vi "EnFlo_Error_Handler.vi"(3 "error in (no error)":errorcluster, 4 "Error Type":string, 5 "Dialog Box (T)":bool=TRUE) -> (0 "Continue":bool, 1 "SMS Message":string, 2 "Email Message":string)   [LabVIEW 2012]
uses:
  Controls/Post_Process.ctl
  <vilib>/Utility/error.llb/DialogType.ctl
  Globals/Meas_global.vi
  Globals/Trav_pos_global.vi
  Globals/Preference_global.vi
  Email_transfer_global.vi
  Globals/Dynamic_call_global.ph.vi
panel:
  out "error out":errorcluster
  in  "Case Constant\n(See Context Help)":bool
  out "Server copy Location":path
  out "Hours Running":dbl format="%.2f"
  out "Raw data file Local":path
  out "Error Information":string
  out "Log Files":path[](array[path])
  out "Frequency":i32
  out "Error Analysis":string
  out "Error Types":string[](array[string])
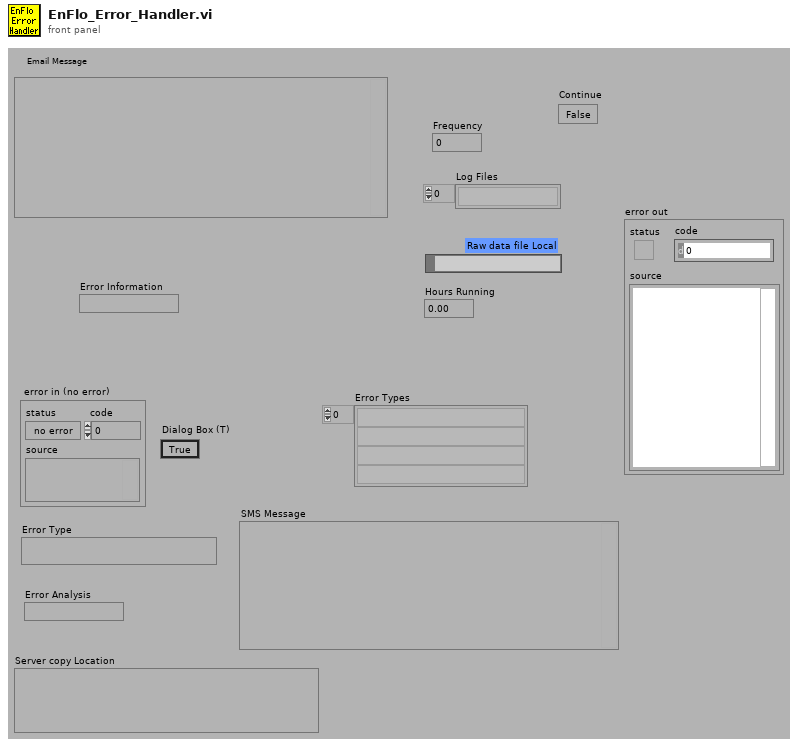
[diagram p1: front panel]
types:
  T1 = typedef "Post_Process.ctl" = enum16{"Take New Data", "Post Process Raw Data File"}
  T2 = cluster{"path":path, "data":string, "binary":bool, "MIME content-type \n(application/octet-stream)":string}[]
  T3 = typedef "DialogType.ctl" = u16
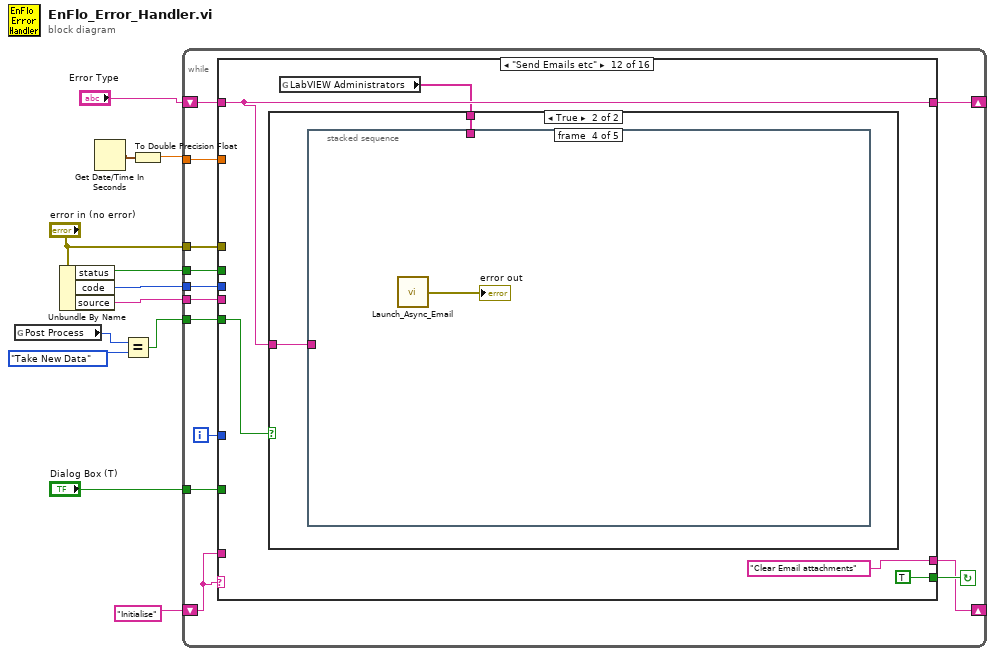
[diagram p0: block diagram]
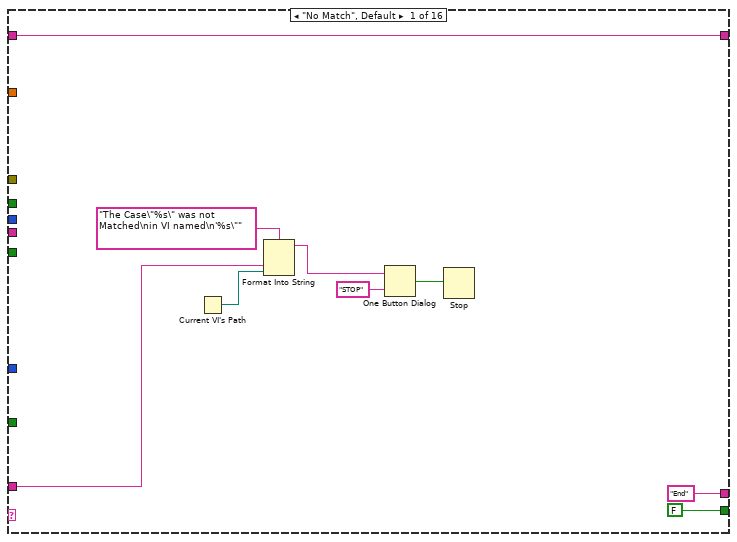
[diagram p2: hidden frame]
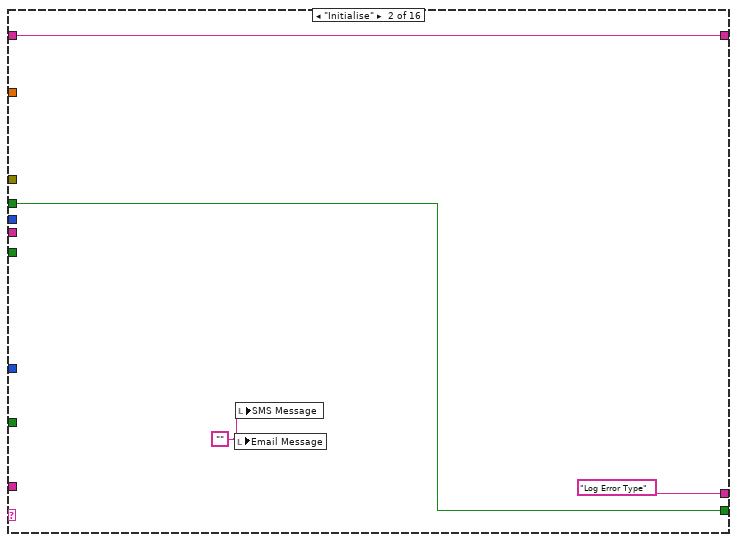
[diagram p3: hidden frame]
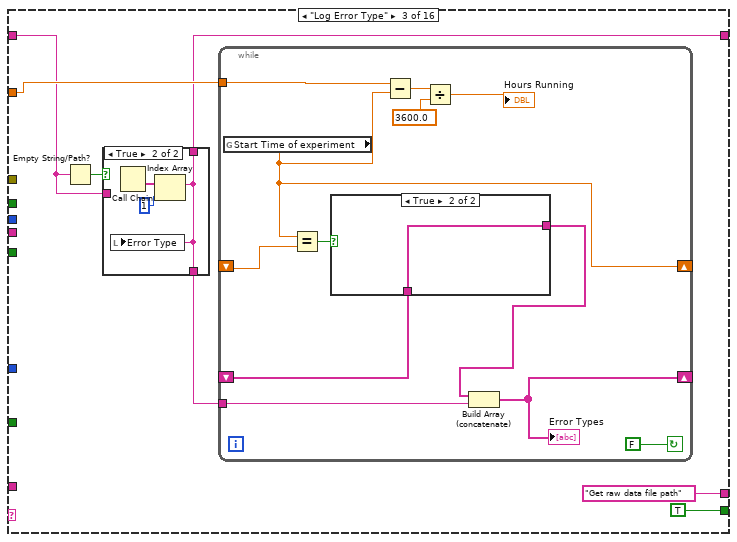
[diagram p4: hidden frame]
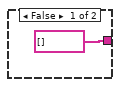
[diagram p5: hidden frame]
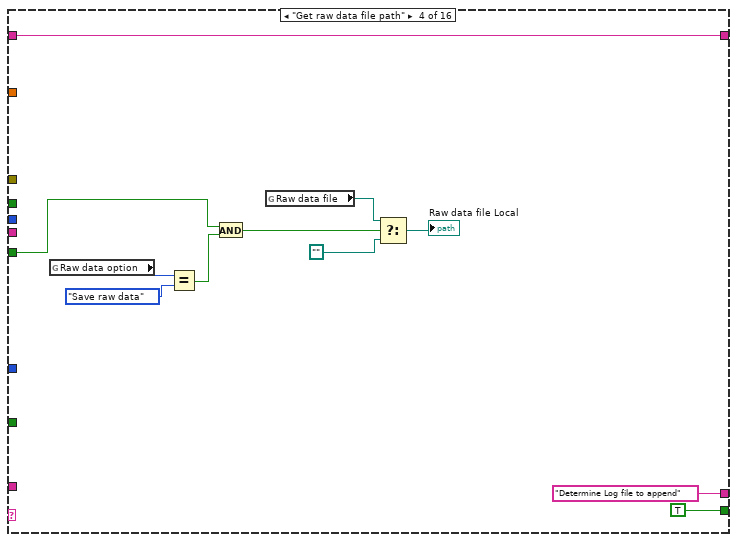
[diagram p7: hidden frame]
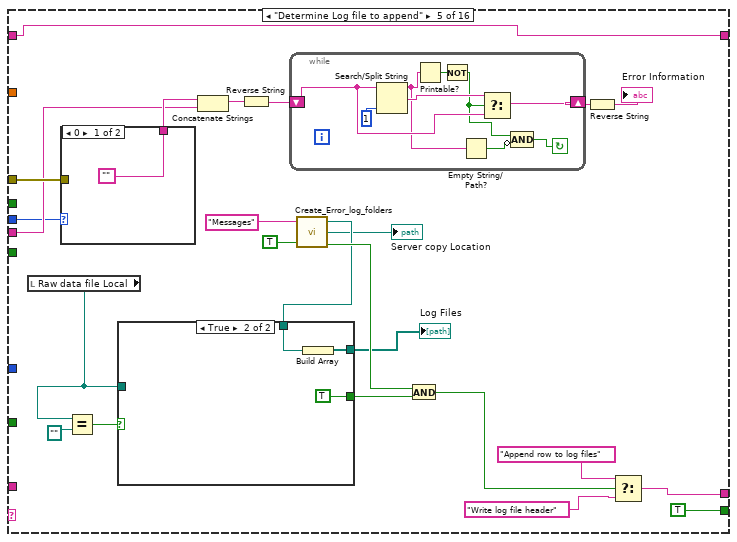
[diagram p8: hidden frame]
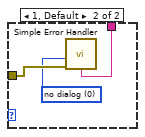
[diagram p9: hidden frame]
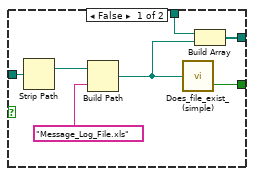
[diagram p10: hidden frame]
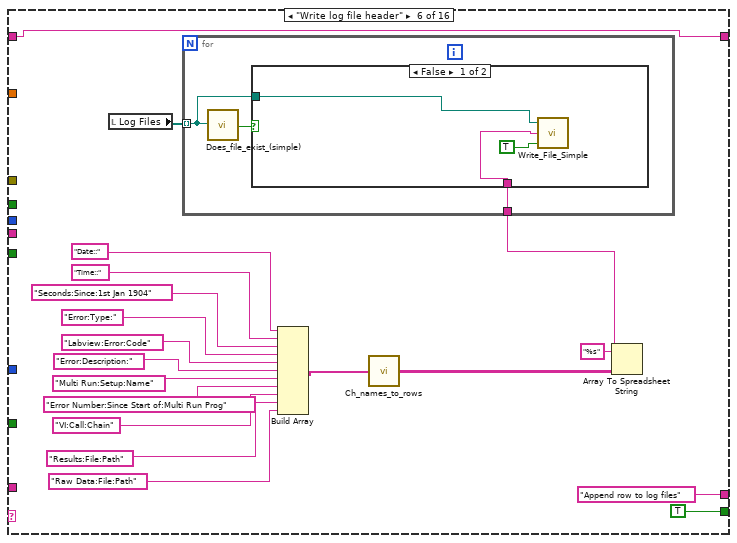
[diagram p11: hidden frame]
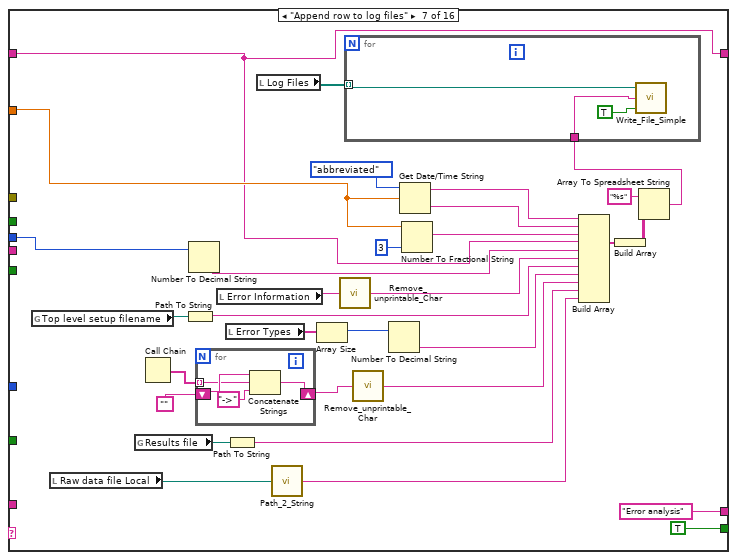
[diagram p13: hidden frame]
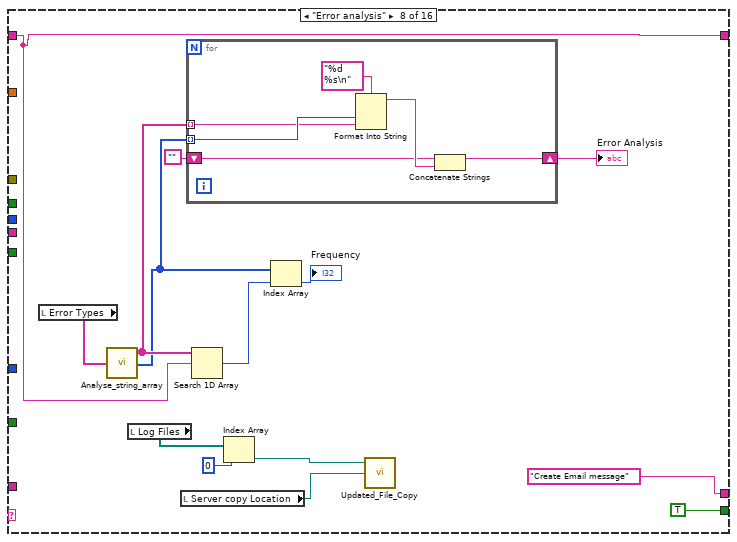
[diagram p14: hidden frame]
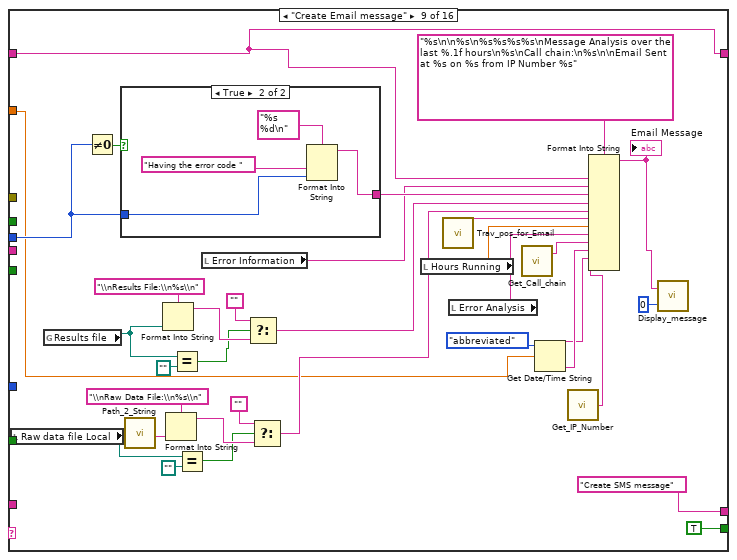
[diagram p15: hidden frame]
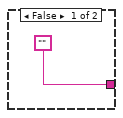
[diagram p16: hidden frame]
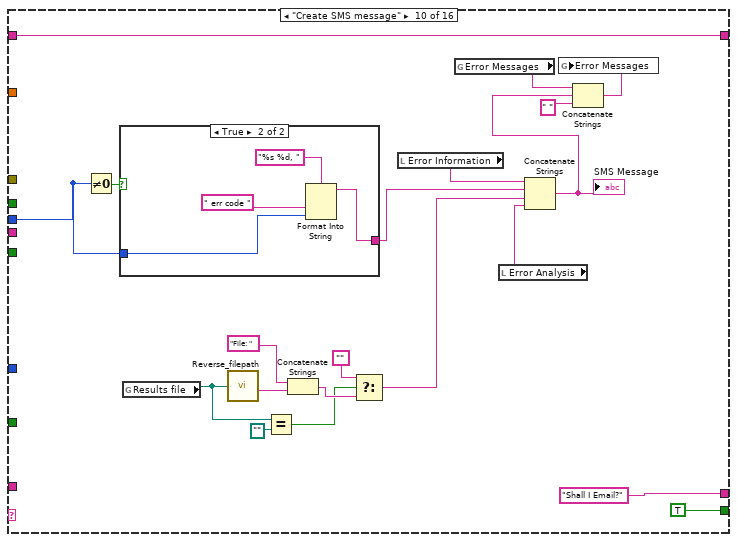
[diagram p17: hidden frame]
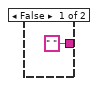
[diagram p18: hidden frame]
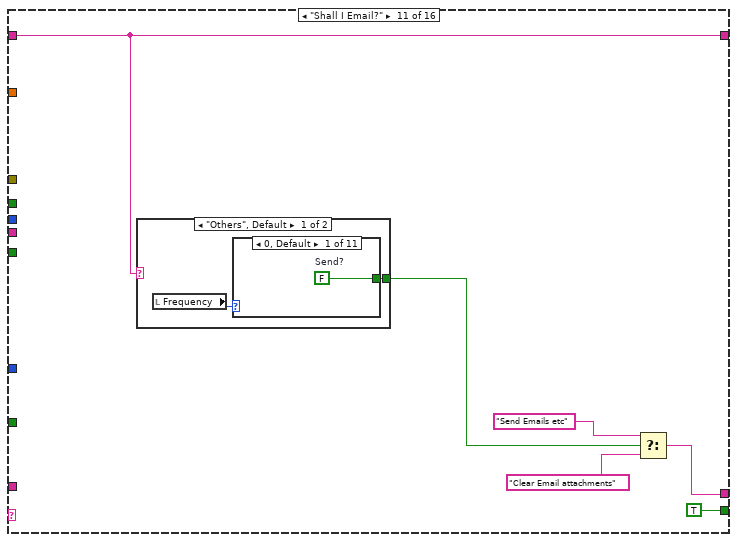
[diagram p19: hidden frame]
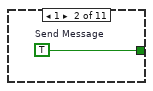
[diagram p20: hidden frame]
diagram:
  n1 = global read "Meas_global.vi" "Post Process"() -> (w5:T1)
  n2 = Unbundle By Name("error in (no error)") -> ("status"=w11:bool, "code"=w10:i32, "source"=w9:string)
  n3 = Get Date/Time In Seconds() -> (seconds since 1Jan1904=w8:timestamp)
  n4 = Equal?(x=w5, y=Post_Process."Take New Data" ("Post Process")) -> (x = y?=w3:bool)
  n5 = To Double Precision Float(number=w8) -> (double precision float=w12:dbl)
  n6 = while {
    tunnel: w9 -> [w19]
    tunnel: w10 -> [w21]
    tunnel: w11 -> [w22]
    tunnel: w12 -> [w23]
    shift-left: "Initialise" -> [w18]
    shift-right: [w24] -> _
    shift-right: [w16] -> _
    shift-left: "Error Type" -> [w17]
    tunnel: w3 -> [w15]
    tunnel: "Dialog Box (T)" -> [w14]
    tunnel: "error in (no error)" -> [w13]
    i -> [w20]
    stop <- w25 continue-if-true
    n7 = case shown="\"Send Emails etc\"" w18 {
      tunnel: [FALSE ("Abort") w38 TRUE ("status") TRUE ("status") TRUE ("status") TRUE TRUE TRUE ("status") TRUE ("Abort") TRUE ("status") TRUE ("Abort") TRUE ("Abort") TRUE ("Abort") w340 w351 FALSE ("Abort")] -> w25
      tunnel: ["End" ("f") "Log Error Type" "Get raw data file path" ("f") "Determine Log file to append" ("f") w96 "Append row to log files" ("f") "Error analysis" ("f") "Create Email message" ("f") "Create SMS message" "Shall I Email?" w272 "Clear Email attachments" "Is ADAM scan table running?" ("f") "Show timed error dialog" "Stop" "End"] -> w24
      tunnel: w23 -> [_ _ w42 _ _ _ w152 _ w215 _ _ _ _ _ _ _]
      tunnel: w22 -> [_ w38 _ _ _ _ _ _ _ _ _ _ _ _ _ _]
      tunnel: w21 -> [_ _ _ _ w75 _ w172 _ w237 w262 _ _ _ _ _ _]
      tunnel: w20 -> [_ _ _ _ _ _ _ _ _ _ _ _ _ _ _ _]
      tunnel: w19 -> [_ _ _ _ w77 _ _ _ _ _ _ _ _ _ _ _]
      tunnel: w18 -> [w29 _ _ _ _ _ _ _ _ _ _ _ _ _ _ _]
      tunnel: w17 -> [w26 w35 w40 w67 w82 w122 w149 w190 w209 w244 w274 w292 w338 w342 w349 w355]
      tunnel: [w26 w35 w39 w67 w82 w122 w149 w190 w209 w244 w274 w292 w338 w342 w349 w355] -> w16
      tunnel: w15 -> [_ _ _ w64 _ _ _ _ _ _ _ w289 _ _ _ _]
      tunnel: w14 -> [_ _ _ _ _ _ _ _ _ _ _ _ _ w339 _ _]
      tunnel: w13 -> [_ _ _ _ w79 _ _ _ _ _ _ _ _ _ _ _]
      frame "No Match", Default {
        n8 = Current VI's Path() -> (path=w30:path)
        n9 = Format Into String(format string="The Case\"%s\" was not Matched\nin VI named\n'%s\"" ("Format String"), w29, w30) -> (resulting string=w33:string)  [unwired: 2 in, 1 out]
        n10 = One Button Dialog(message=w33, button name ("OK")="STOP") -> (true=w31:bool)
        n11 = Stop(stop? (T)=w31) -> ()
      }
      frame "Initialise" {
        w37 = ""
        n12 = local write "Email Message"(w37) -> ()
        n13 = local write "SMS Message"(w37) -> ()
      }
      frame "Log Error Type" {
        n14 = Empty String/Path?(string/path=w40) -> (empty?=w44:bool)
        n15 = case shown="True" w44 {
          tunnel: [w60 w61] -> w43
          tunnel: w40 -> [w60 _]
          tunnel: [w60 w61] -> w39
          frame False {
          }
          frame True {
            n16 = Call Chain() -> (call chain=w63:string[])
            n17 = Index Array(array=w63, index=1 ("Index")) -> (element=w61:string)
            n18 = local write "Error Type"(w61) -> ()
          }
        }
        n19 = while {
          tunnel: w42 -> [w48]
          shift-left: _ -> [w55]
          shift-right: [w54] -> _
          shift-left: _ -> [w53]
          shift-right: [w51] -> _
          tunnel: w43 -> [w56]
          stop <- FALSE continue-if-true
          n20 = global read "Meas_global.vi" "Start Time of experiment"() -> (w51:dbl)
          n21 = Equal?(x=w51, y=w53) -> (x = y?=w52:bool)
          n22 = case shown="True" w52 {
            tunnel: [string[] [] w59] -> w57
            tunnel: w55 -> [_ w59]
            frame False {
            }
            frame True {
            }
          }
          n23 = Subtract(x=w48, y=w51) -> (x-y=w50:dbl)
          n24 = Divide(x=w50, y=3600.0) -> (x/y=→"Hours Running":dbl)
          n25 = Build Array (concatenate)(w57, w56) -> (w54:string[])
          "Error Types" <- w54
        }
      }
      frame "Get raw data file path" {
        n26 = global read "Meas_global.vi" "Raw data option"() -> (w73:enum16{"Save raw data", "Raw data not saved"})
        n27 = Equal?(x=w73, y=enum16{"Save raw data", "Raw data not saved"}."Save raw data" ("Raw data option")) -> (x = y?=w71:bool)
        n28 = And(x=w64, y=w71) -> (x .and. y?=w70:bool)
        n29 = global read "Meas_global.vi" "Raw data file"() -> (w66:path)
        n30 = Select(t=w66, s=w70, f=path "") -> (s? t:f=→"Raw data file Local":path)
      }
      frame "Determine Log file to append" {
        n31 = local read "Raw data file Local"() -> (w85:path)
        n32 = case shown="0" w75 {
          tunnel: w79 -> [_ w102]
          tunnel: ["" w100] -> w78
          frame 0 {
          }
          frame 1, Default {
            w101 = T3 0 items=["no dialog", "OK message", "continue or stop message", "OK message + warnings", "continue/stop + warnings"] ("type of dialog (OK msg:1)")
            n33 = call <vilib>:"Simple Error Handler.vi"("type of dialog (OK msg:1)"=w101, "error in (no error)"=w102) -> ("message"=w100:string)  [unwired: 7 out]
          }
        }
        n34 = Equal?(x=w85, y=path "") -> (x = y?=w94:bool)
        n35 = Concatenate Strings(w78, w77) -> (w76:string)
        n36 = Reverse String(1:w76) -> (0:w88:string)
        n37 = while {
          shift-left: w88 -> [w109]
          shift-right: [w108] -> w87
          stop <- w103 continue-if-true
          n38 = Search/Split String(string=w109, offset (0)=1 ("length")) -> (substring before match=w106:string, match + rest of string=w110:string)  [unwired: 2 out]
          n39 = Printable?(1:w106) -> (0:w107:bool)
          n40 = Not(x=w107) -> (.not. x?=w105:bool)
          n41 = Empty String/Path?(string/path=w106) -> (empty?=w104:bool)
          n42 = Select(t=w110, s=w105, f=w109) -> (s? t:f=w108:string)
          n43 = Compound Arithmetic op=AND(w105, invert w104) -> (w103:bool)
        }
        n44 = call "Create_Error_log_folders.vi"("Per Day Log File?"=TRUE, "Log Filename"="Messages" ("Input Element")) -> ("exists?"=w92:bool, "Server copy Location"=→"Server copy Location":path, "Local Log File"=w90:path)  [unwired: 1 in]
        n45 = case shown="True" w94 {
          tunnel: w85 -> [w118 _]
          tunnel: [w115 TRUE ("exists?")] -> w93
          tunnel: w90 -> [w114 w120]
          tunnel: [w112 w119] -> w89
          frame False {
            n46 = Strip Path(path=w118) -> (stripped path=w117:path)  [unwired: 1 out]
            n47 = Build Path(base path=w117, name or relative path="Message_Log_File.xls") -> (appended path=w113:path)
            n48 = call "Does_file_exist_(simple).vi"("Pathname"=w113) -> ("exists?"=w115:bool)
            n49 = Build Array(w114, w113) -> (w112:path[])
          }
          frame True {
            n50 = Build Array(w120) -> (w119:path[])
          }
        }
        "Log Files" <- w89
        n51 = And(x=w92, y=w93) -> (x .and. y?=w91:bool)
        n52 = Reverse String(1:w87) -> (0:→"Error Information":string)
        n53 = Select(t="Append row to log files", s=w91, f="Write log file header") -> (s? t:f=w96:string)
      }
      frame "Write log file header" {
        n54 = local read "Log Files"() -> (w126:path[])
        n55 = Build Array("Date::", "Time::", "Seconds:Since:1st Jan 1904", "Error:Type:", "Labview:Error:Code", "Error:Description:", "Multi Run:Setup:Name", "Error Number:Since Start of:Multi Run Prog", "VI:Call:Chain", "Results:File:Path", "Raw Data:File:Path") -> (w125:string[])
        n56 = call "Ch_names_to_rows.vi"("Channel Names"=w125) -> ("3 Row names"=w124:string[][])
        n57 = Array To Spreadsheet String(array=w124, 3:"%s" ("format string")) -> (spreadsheet string=w130:string)  [unwired: 1 out]
        n58 = for {
          tunnel: w130 -> [w143]
          tunnel: w126 -> [w141] mode=indexing
          n59 = call "Does_file_exist_(simple).vi"("Pathname"=w141) -> ("exists?"=w142:bool)
          n60 = case shown="False" w142 {
            tunnel: w143 -> [w145 _]
            tunnel: w141 -> [w144 _]
            frame False {
              n61 = call "Write_File_Simple.vi"("append to file? (new file:F)"=TRUE, "character string"=w145, "file path"=w144) -> ()  [unwired: 2 out]
            }
            frame True {
            }
          }
        }
      }
      frame "Append row to log files" {
        n62 = global read "Trav_pos_global.vi" "Top level setup filename"() -> (w174:path)
        n63 = local read "Raw data file Local"() -> (w148:path)
        n64 = global read "Meas_global.vi" "Results file"() -> (w157:path)
        n65 = Call Chain() -> (call chain=w162:string[])
        n66 = Path To String(path=w174) -> (string=w169:string)
        n67 = Number To Decimal String(number=w172) -> (decimal integer string=w171:string)  [unwired: 1 out]
        n68 = for {
          shift-right: [w181] -> w161
          shift-left: "" -> [w184]
          tunnel: w162 -> [w183] mode=indexing
          n69 = Concatenate Strings(w184, w183, "->" ("Substring")) -> (w181:string)
        }
        n70 = local read "Error Information"() -> (w154:string)
        n71 = local read "Error Types"() -> (w167:string[])
        n72 = Path To String(path=w157) -> (string=w156:string)
        n73 = local read "Log Files"() -> (w155:path[])
        n74 = call "Path_2_String.vi"("Real Path"=w148) -> ("Path String"=w147:string)
        n75 = Array Size(array=w167) -> (size(s)=w173:i32)
        n76 = call "Remove_unprintable_Char.vi"("Input String"=w154) -> ("Output String"=w170:string)
        n77 = call "Remove_unprintable_Char.vi"("Input String"=w161) -> ("Output String"=w163:string)
        n78 = Number To Decimal String(number=w173) -> (decimal integer string=w168:string)  [unwired: 1 out]
        n79 = Get Date/Time String(date format (0)=enum16{"short", "long", "abbreviated"}."abbreviated", seconds (now)=w152) -> (date string=w176:string, time string=w175:string)  [unwired: 1 out]
        n80 = Number To Fractional String(number=w152, precision (6)=i16 3) -> (F-format string=w151:string)  [unwired: 2 out]
        n81 = Build Array(w176, w175, w151, w149, w171, w170, w169, w168, w163, w156, w147) -> (w158:string[])
        n82 = Build Array(w158) -> (w166:string[][])
        n83 = Array To Spreadsheet String(array=w166, 3:"%s" ("format string")) -> (spreadsheet string=w164:string)  [unwired: 1 out]
        n84 = for {
          tunnel: w164 -> [w179]
          tunnel: w155 -> [w178] mode=indexing
          n85 = call "Write_File_Simple.vi"("append to file? (new file:F)"=TRUE, "character string"=w179, "file path"=w178) -> ()  [unwired: 2 out]
        }
      }
      frame "Error analysis" {
        n86 = local read "Error Types"() -> (w193:string[])
        n87 = call "Analyse_string_array.vi"("String array"=w193) -> ("Unique strings"=w197:string[], "Frequency"=w196:i32[])  [unwired: 1 out]
        n88 = local read "Log Files"() -> (w188:path[])
        n89 = local read "Server copy Location"() -> (w185:path)
        n90 = for {
          tunnel: w197 -> [w202] mode=indexing
          tunnel: w196 -> [w203] mode=indexing
          shift-right: [w199] -> w194
          shift-left: "" -> [w200]
          n91 = Format Into String(format string="%d %s\n" ("Format String"), w203, w202) -> (resulting string=w201:string)  [unwired: 2 in, 1 out]
          n92 = Concatenate Strings(w200, w201) -> (w199:string)
        }
        "Error Analysis" <- w194
        n93 = Search 1D Array(1D array=w197, element=w190) -> (index of element=w198:i32)  [unwired: 1 out]
        n94 = Index Array(array=w188, index=0) -> (element=w186:path)
        n95 = Index Array(array=w196, index=w198) -> (element=→"Frequency":i32)
        n96 = call "Updated_File_Copy.vi"("Target Path"=w185, "Source Path"=w186) -> ()  [unwired: 2 out]
      }
      frame "Create Email message" {
        n97 = local read "Raw data file Local"() -> (w206:path)
        n98 = global read "Meas_global.vi" "Results file"() -> (w222:path)
        n99 = Not Equal To 0?(x=w237) -> (x != 0?=w238:bool)
        n100 = case shown="True" w238 {
          tunnel: w237 -> [_ w242]
          tunnel: ["" w240] -> w236
          frame False {
          }
          frame True {
            n101 = Format Into String(format string="%s %d\n" ("Format String"), "Having the error code ", w242) -> (resulting string=w240:string)  [unwired: 2 in, 1 out]
          }
        }
        n102 = call "Path_2_String.vi"("Real Path"=w206) -> ("Path String"=w205:string)
        n103 = Format Into String(format string="\\nResults File:\\n%s\\n" ("Format String"), w222) -> (resulting string=w228:string)  [unwired: 2 in, 1 out]
        n104 = Format Into String(format string="\\nRaw Data File:\\n%s\\n" ("Format String"), w205) -> (resulting string=w226:string)  [unwired: 2 in, 1 out]
        n105 = Equal?(x=w222, y=path "") -> (x = y?=w221:bool)
        n106 = Equal?(x=w206, y=path "") -> (x = y?=w223:bool)
        n107 = local read "Error Information"() -> (w220:string)
        n108 = Select(t="", s=w221, f=w228) -> (s? t:f=w231:string)
        n109 = Select(t="", s=w223, f=w226) -> (s? t:f=w230:string)
        n110 = local read "Hours Running"() -> (w218:dbl)
        n111 = call "Trav_pos_for_Email.vi"() -> ("String"=w219:string)
        n112 = local read "Error Analysis"() -> (w217:string)
        n113 = call "Get_Call_chain.vi"() -> ("Output String"=w216:string)  [unwired: 1 in, 1 out]
        n114 = Get Date/Time String(date format (0)=enum16{"short", "long", "abbreviated"}."abbreviated", seconds (now)=w215) -> (date string=w211:string, time string=w213:string)  [unwired: 1 out]
        n115 = call "Get_IP_Number.vi"() -> ("IP Number"=w207:string)
        n116 = Format Into String(format string="%s\n\n%s\n%s%s%s%s\nMessage Analysis over the last %.1f hours\n%s\nCall chain:\n%s\n\nEmail Sent at %s on %s from IP Number %s" ("Format String"), w209, w220, w236, w231, w230, w219, w218, w217, w216, w213, w211, w207) -> (resulting string=w212:string)  [unwired: 2 in, 1 out]
        "Email Message" <- w212
        n117 = call "Display_message.vi"("Time to display message"=u32 0, "Message"=w212) -> ()  [unwired: 2 out]
      }
      frame "Create SMS message" {
        n118 = Not Equal To 0?(x=w262) -> (x != 0?=w263:bool)
        n119 = case shown="True" w263 {
          tunnel: w262 -> [_ w267]
          tunnel: [" " w265] -> w261
          frame False {
          }
          frame True {
            n120 = Format Into String(format string="%s %d, " ("Format String"), " err code ", w267) -> (resulting string=w265:string)  [unwired: 2 in, 1 out]
          }
        }
        n121 = global read "Meas_global.vi" "Results file"() -> (w248:path)
        n122 = call "Reverse_filepath.vi"("Filename"=w248) -> ("Reversed Filepath"=w255:string)
        n123 = Equal?(x=w248, y=path "") -> (x = y?=w247:bool)
        n124 = Concatenate Strings("File: ", w255) -> (w253:string)
        n125 = Select(t="", s=w247, f=w253) -> (s? t:f=w251:string)
        n126 = local read "Error Information"() -> (w246:string)
        n127 = global read "Meas_global.vi" "Error Messages"() -> (w258:string)
        n128 = local read "Error Analysis"() -> (w250:string)
        n129 = Concatenate Strings(w246, w261, w251, w250) -> (w256:string)
        "SMS Message" <- w256
        n130 = Concatenate Strings(w258, w256, " ") -> (w257:string)
        n131 = global write "Meas_global.vi" "Error Messages"(w257) -> ()
      }
      frame "Shall I Email?" {
        n132 = case shown="\"Others\", Default" w274 {
          tunnel: [w275 TRUE ("Send Message")] -> w273
          frame "Others", Default {
            n133 = local read "Frequency"() -> (w276:i32)
            n134 = case shown="0, Default" w276 {
              tunnel: [w277 w278 w279 w280 TRUE TRUE TRUE TRUE TRUE TRUE w287] -> w275
              frame 0, Default {
                w277 = FALSE  # Send?
              }
              frame 1 {
                w278 = TRUE  # Send Message
              }
              frame 2 {
                w279 = TRUE  # Send Message
              }
              frame 5 {
                w280 = TRUE  # Send Message
              }
              frame 10 {
              }
              frame 20 {
              }
              frame 50 {
              }
              frame 100 {
              }
              frame 200 {
              }
              frame 500 {
              }
              frame 1000 {
                w287 = TRUE  # Send Message
              }
            }
          }
          frame "Message" {
          }
        }
        n135 = Select(t="Send Emails etc", s=w273, f="Clear Email attachments") -> (s? t:f=w272:string)
      }
      frame "Send Emails etc" {
        n136 = global read "Preference_global.vi" "LabVIEW Administrators"() -> (w290:string[])
        n137 = case shown="True" w289 {
          tunnel: w292 -> [_ w295]
          tunnel: w290 -> [_ w294]
          frame False {
          }
          frame True {
            n138 = stacked-sequence {
              tunnel: w295 -> [_ w300 _ _ w322]
              tunnel: w294 -> [w297 _ w314 _ _]
              frame #0 {
                n139 = global read "Meas_global.vi" "People to Email"() -> (w296:string[])
                n140 = global read "Email_transfer_global.vi" "recipients"() -> (w298:string[])
                n141 = Build Array (concatenate)(w298, w297, w296) -> (w299:string[])
                n142 = global write "Email_transfer_global.vi" "recipients"(w299) -> ()
              }
              frame #1 {
                n143 = global write "Email_transfer_global.vi" "subject ([No Subject])"(w300) -> ()
              }
              frame #2 {
                n144 = local read "Email Message"() -> (w301:string)
                n145 = Concatenate Strings(w301, "\nThis email has been generated  automatically by LabVIEW. If you need help with understanding the email, or want to be removed from the mailing list please contact:\n") -> (w312:string)
                n146 = Concatenate Strings(" or ", "\r\n") -> (w308:string)
                n147 = for {
                  shift-right: [w316] -> w311
                  shift-left: w312 -> [w318]
                  tunnel: w314 -> [w317] mode=indexing
                  tunnel: w308 -> [w315]
                  n148 = Concatenate Strings(w318, w317, w315) -> (w316:string)
                }
                n149 = String Length(string=w308) -> (length=w306:i32)
                n150 = String Length(string=w311) -> (length=w307:i32)
                n151 = Subtract(x=w307, y=w306) -> (x-y=w305:i32)
                n152 = String Subset(string=w311, length (rest)=w305) -> (substring=w304:string)  [unwired: 1 out]
                n153 = Concatenate Strings(w304, "\r\n") -> (w302:string)
                n154 = global write "Email_transfer_global.vi" "message"(w302) -> ()
              }
              frame #3 {
                n155 = call "Launch_Async_Email.vi"() -> ("error out"=→"error out":errorcluster)  [unwired: 2 out]
              }
              frame #4 {
                n156 = local read "Frequency"() -> (w320:i32)
                n157 = case shown="\"No Match\", Default" w322 {
                  tunnel: [TRUE FALSE w330 FALSE] -> w324
                  tunnel: w320 -> [_ _ w332 _]
                  frame "No Match", Default {
                  }
                  frame "Pulse Width Error" {
                  }
                  frame "LDA Invalid Bursts" {
                    n158 = Greater?(x=w332, y=4) -> (0:w330:bool)
                  }
                  frame "Warning" {
                  }
                }
                n159 = global read "Meas_global.vi" "People to Email"() -> (w321:string[])
                n160 = local read "SMS Message"() -> (w323:string)
                n161 = case shown="True" w324 {
                  tunnel: w323 -> [_ w327]
                  tunnel: w321 -> [_ w326]
                  tunnel: w322 -> [_ w325]
                  frame False {
                  }
                  frame True {
                    n162 = call "SMS_to_mobile.vi"("SMS address"=w326, "Subject"=w325, "Message"=w327) -> ()  [unwired: 3 out]
                  }
                }
              }
            }
          }
        }
      }
      frame "Clear Email attachments" {
        n163 = global write "Email_transfer_global.vi" "attachments"(T2 [] ("attachments")) -> ()
        n164 = global write "Email_transfer_global.vi" "recipients"(string[] [] ("recipients")) -> ()
      }
      frame "Is ADAM scan table running?" {
        n165 = Open VI Reference(vi path="ADAM_scan_table.vi") -> (vi reference=w346:refnum<vi>, error out=w345:errorcluster)  [unwired: 1 in, 4 out]
        n166 = Unbundle By Name(w345) -> ("status"=w341:bool)
        n167 = case shown="False" w341 {
          tunnel: w345 -> [w348 _]
          tunnel: w346 -> [w347 _]
          frame False {
            n168 = Close Reference(reference=w347, error in (no error)=w348) -> ()  [unwired: 1 out]
          }
          frame True {
          }
        }
        n169 = Compound Arithmetic op=AND(w341, w339) -> (w340:bool)
      }
      frame "Show timed error dialog" {
        n170 = local read "Email Message"() -> (w353:string)
        n171 = call "Timed_Error_dialog.vi"("Message"=w353, "Seconds to wait"=60.0) -> ("Ignore"=→"Continue":bool, "Abort"=w351:bool)
      }
      frame "Stop" {
        n172 = stacked-sequence {
          seq-local: [_ w365 _ _ _] -> [_ _ w379 _ _]
          frame #0 {
            n173 = call "Program_Active_Aborting.vi"() -> ()  [unwired: 6 out]
          }
          frame #1 {
            n174 = Build Array("Edit_BSA_setup.vi", "Measurement_input_panel.vi", "Input_Value_Dialog.vi", "Input_String_Dialog.vi", "Calibration_user_input.vi", "Input_Traverse_position.vi", "User_Metadata.vi", "Preference_Panel.vi", "Traverse_Space.vi", "Enter_Temp_Press.vi", "EnFlo_Tunnel_Setup.vi", "Gas_Setup.vi", "Correlation_Display.vi", "Serial_Setup.vi", "Port_Names.vi", "Select_Strings.vi", "Edit_Template_File.vi", "Select_a_Channel.vi", "Output_file_Panel.vi", "Enter_LDA_Setup.vi") -> (w365:string[])
          }
          frame #2 {
            n175 = for {
              tunnel: w379 -> [w380] mode=indexing
              n176 = Open VI Reference(vi path=w380) -> (vi reference=w385:refnum<vi>, error out=w384:errorcluster)  [unwired: 1 in, 4 out]
              n177 = property class="VI"(reference=w385, error in=w384, "Front Panel Window:Open"=FALSE) -> (reference out=w383:refnum<vi>, error out=w382:errorcluster)
              n178 = Close Reference(reference=w383, error in (no error)=w382) -> ()  [unwired: 1 out]
            }
          }
          frame #3 {
            n179 = case shown="True" "Case Constant\n(See Context Help)" {
              frame False {
              }
              frame True {
                # "Cased out 4/7/07 because it hung code"
                n180 = global write "Dynamic_call_global.ph.vi" "EnFlo Hub running?"(FALSE ("EnFlo Hub running?")) -> ()
              }
            }
          }
          frame #4 {
            n181 = Stop(stop? (T)=TRUE) -> ()
          }
        }
      }
    }
  }
